vi "Deadband Calculation.vi"(6 "Min Deadband":dbl, 7 "Max Deadband":dbl, 11 "Deadband Check Input":dbl) -> (3 "Deadband Check Output":dbl)   [LabVIEW 2017]
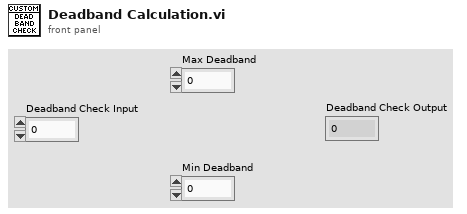
[diagram p1: front panel]
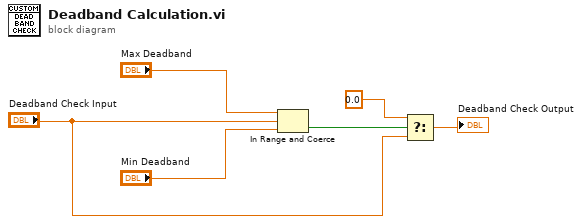
[diagram p0: block diagram]
diagram:
  n1 = In Range and Coerce(upper limit="Max Deadband", x="Deadband Check Input", lower limit="Min Deadband") -> (In Range?=w4:bool)  [unwired: 1 out]
  n2 = Select(t=0.0, s=w4, f="Deadband Check Input") -> (s? t:f=→"Deadband Check Output":dbl)
